vi "SetOutputVoltage_online.vi"() -> ()   [LabVIEW 2018]
uses:
  <vilib>/Utility/error.llb/DialogType.ctl
  <vilib>/DAQmx/write.llb/DAQmx Write (Analog 2D DBL NChan NSamp).vi
  <vilib>/DAQmx/create/channels.llb/DAQmx Create Channel (AO-Voltage-Basic).vi
  <vilib>/DAQmx/configure/timing.llb/DAQmx Timing (Sample Clock).vi
  <vilib>/DAQmx/configure/trigger.llb/DAQmx Start Trigger (Digital Edge).vi
  <vilib>/DAQmx/configure/trigger.llb/DAQmx Start Trigger (Time).vi
  <vilib>/DAQmx/configure/trigger.llb/DAQmx Start Trigger (Analog Edge).vi
  <vilib>/DAQmx/miscellaneous.llb/DAQmx Fill In Error Info.vi
  <resource>/objmgr/daqmx.rc
panel:
  in  "element":dbl=0.1 format="%#_13g"
  in  "Trigger Type":T1(tab)
  in  "Digital Start Trigger Edge":i32(ring)=10280 caption="Edge" items=["Rising"=10280, "Falling"=10171]
  in  "Digital Start Trigger Source":tag="/Dev1/PFI0" caption="Source"
  in  "Digital Pause Trigger Pause When":i32(ring)=10192 caption="Pause When" items=["High"=10192, "Low"=10214]
  in  "Digital Pause Trigger Source":tag="/Dev1/PFI0" caption="Source"
  in  "Analog Start Trigger Level":dbl caption="Level" format="%0.2f"
  in  "Analog Start Trigger Hysteresis":dbl caption="Hysteresis" format="%.2f"
  in  "Analog Start Trigger Slope":i32(ring)=10280 caption="Slope" items=["Rising"=10280, "Falling"=10171]
  in  "Analog Start Trigger Source":string="APFI0" caption="Source"
  in  "Analog Pause Trigger Source":string="APFI0" caption="Source"
  in  "Analog Pause Trigger Pause When":i32(ring)=10093 caption="Pause When" items=["Above Level"=10093, "Below Level"=10107]
  in  "Analog Pause Trigger Level":dbl caption="Level" format="%.2f"
  in  "When":timestamp
  in  "Select Time\nManually":bool
  out "Waveform Graph":waveform(dbl)[](graph)=[{"t0"=timestamp(0 s since 1904-01-01), "dt"=0.001, "Y"=[]}]
  in  "Stop":bool
  in  "Sample Rate":dbl=1000.0
  in  "Sample Clock Source":tag="OnboardClock"
  in  "Max Voltage":dbl=5.0
  in  "Min Voltage":dbl=-5.0
  in  "Physical Channel(s)":tag="Mod2/ao0"
  out "Actual Sample Rate":dbl=1000.0 format="%0.2f"
  # "To enable triggers, select a tab above, and configure the settings.\n\nNot all hardware supports all trigger types. Refer to your device documentation for more information."
  # "This trigger type is not supported in output tasks. \n\nRefer to your device documentation for more information on which triggers are supported."
  # "This trigger type is not supported in output tasks. \n\nRefer to your device documentation for more information on which triggers are supported."
  # "If time is not manually set, task will begin after 10 seconds"
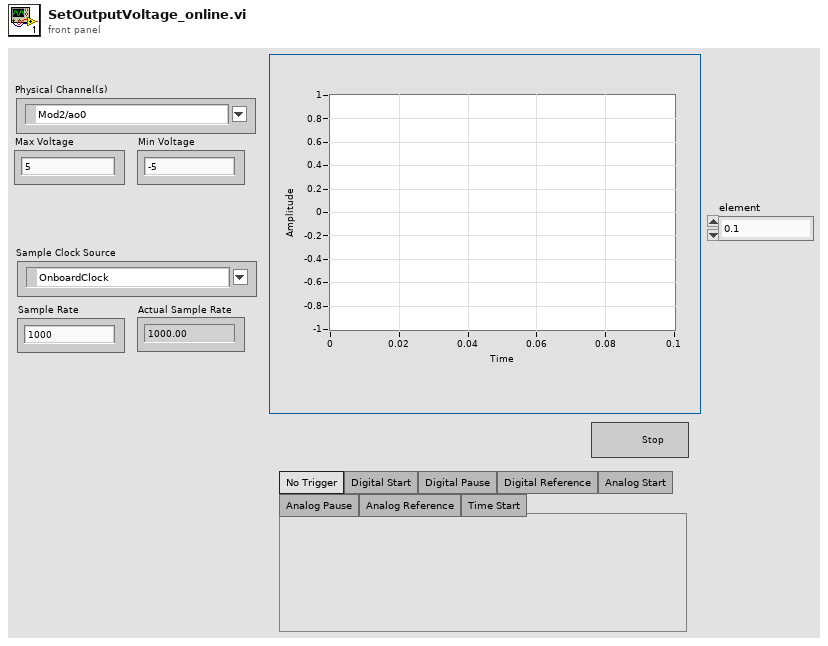
[diagram p1: front panel]
types:
  T1 = enum32{"No Trigger", "Digital Start", "Digital Pause", "Digital Reference", "Analog Start", "Analog Pause", "Analog Reference", "Time Start"}
  T2 = typedef "DialogType.ctl" = u16
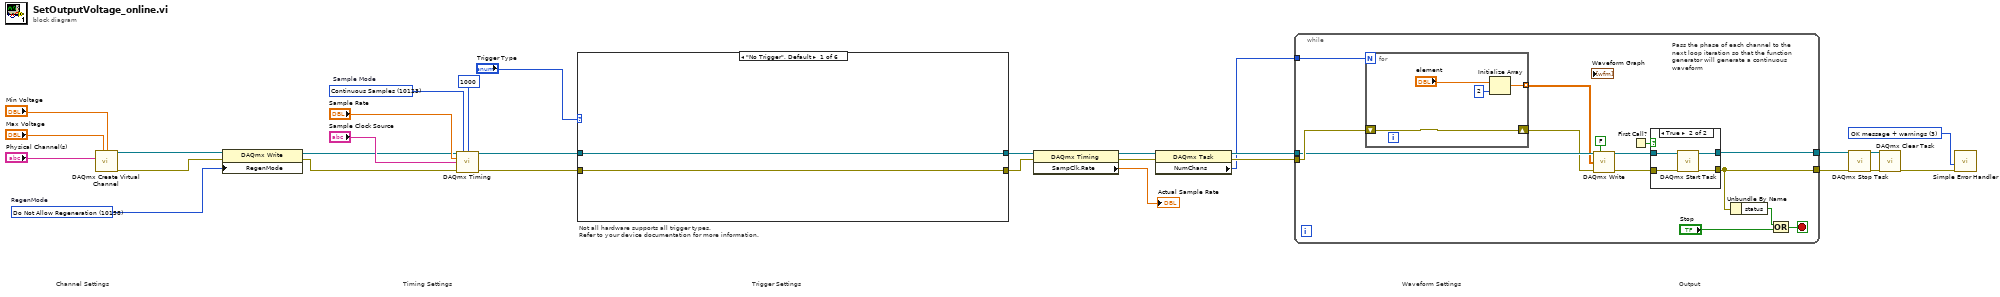
[diagram p0: block diagram]
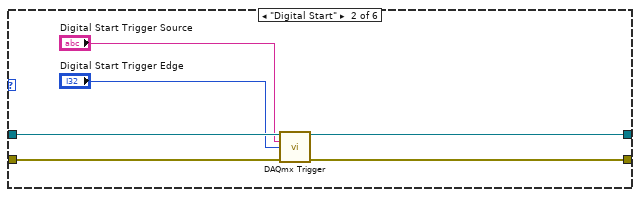
[diagram p3: hidden frame]
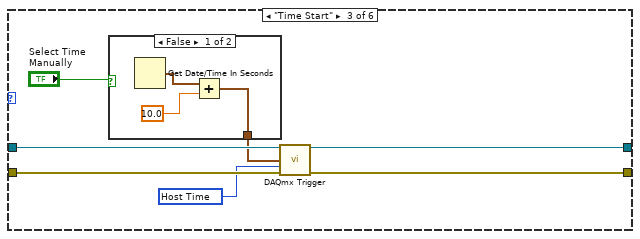
[diagram p4: hidden frame]
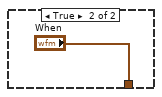
[diagram p5: hidden frame]
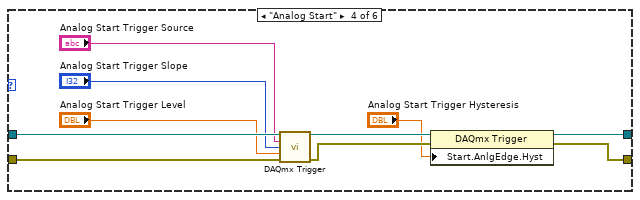
[diagram p6: hidden frame]
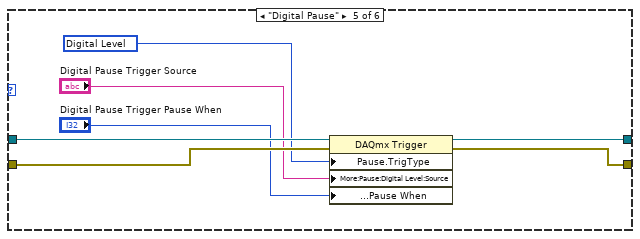
[diagram p7: hidden frame]
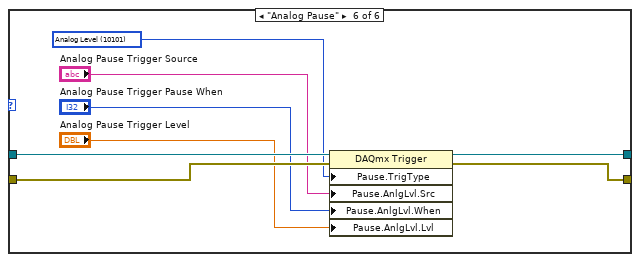
[diagram p8: hidden frame]
diagram:
  w12 = T2 3 items=["no dialog", "OK message", "continue or stop message", "OK message + warnings", "continue/stop + warnings"] ("type of dialog (OK msg:1)")
  w19 = 10158 items=["Allow Regeneration"=10097, "Do Not Allow Regeneration"=10158]  # RegenMode
  w29 = 10123 items=["Finite Samples"=10178, "Continuous Samples"=10123, "Hardware Timed Single Point"=12522]  # Sample Mode
  # "Trigger Settings"
  # "Not all hardware supports all trigger types.\nRefer to your device documentation for more information."
  # "Output"
  # "Waveform Settings"
  # "Timing Settings"
  # "Channel Settings"
  n1 = call-poly <vilib>:"DAQmx Create Virtual Channel.vi"("maximum value"="Max Voltage", "minimum value"="Min Voltage", "physical channels"="Physical Channel(s)") -> ("task out"=w21:refnum<k21>, "error out"=w20:errorcluster)  [unwired: 11 in]
  n2 = property class="DAQmx Write"(reference=w21, error in=w20, "RegenMode"=w19) -> (reference out=w17:refnum<k21>, error out=w18:errorcluster)
  n3 = call-poly <vilib>:"DAQmx Timing.vi"("task/channels in"=w17, "sample mode"=w29, "samples per channel"=1000, "rate"="Sample Rate", "source"="Sample Clock Source", "error in"=w18) -> ("task out"=w5:refnum<k21>, "error out"=w6:errorcluster)  [unwired: 8 in]
  n4 = case shown="\"No Trigger\", Default" "Trigger Type" {
    tunnel: w5 -> [w31 w37 w44 w58 w65 w73]
    tunnel: w6 -> [w30 w36 w43 w57 w62 w70]
    tunnel: [w31 w35 w42 w55 w64 w72] -> w4
    tunnel: [w30 w34 w41 w54 w63 w71] -> w3
    frame "No Trigger", Default {
    }
    frame "Digital Start" {
      n5 = call-poly <vilib>:"DAQmx Trigger.vi"("task/channels in"=w37, "source"="Digital Start Trigger Source", "edge"="Digital Start Trigger Edge", "error in"=w36) -> ("task out"=w35:refnum<k21>, "error out"=w34:errorcluster)  [unwired: 10 in]
    }
    frame "Time Start" {
      w38 = 16126 items=["Host Time"=16126, "I/O Device Time"=16127] ("timescale")
      n6 = case shown="False" "Select Time\nManually" {
        tunnel: [w46 "When"] -> w39
        frame False {
          n7 = Get Date/Time In Seconds() -> (seconds since 1Jan1904=w47:timestamp)
          n8 = Add(x=w47, y=10.0) -> (x+y=w46:timestamp)
        }
        frame True {
        }
      }
      n9 = call-poly <vilib>:"DAQmx Trigger.vi"("task/channels in"=w44, "when"=w39, "timescale"=w38, "error in"=w43) -> ("task out"=w42:refnum<k21>, "error out"=w41:errorcluster)  [unwired: 10 in]
    }
    frame "Analog Start" {
      n10 = call-poly <vilib>:"DAQmx Trigger.vi"("task/channels in"=w58, "source"="Analog Start Trigger Source", "slope"="Analog Start Trigger Slope", "level"="Analog Start Trigger Level", "error in"=w57) -> ("task out"=w53:refnum<k21>, "error out"=w52:errorcluster)  [unwired: 9 in]
      n11 = property class="DAQmx Trigger"(reference=w53, error in=w52, "Start.AnlgEdge.Hyst"="Analog Start Trigger Hysteresis") -> (reference out=w55:refnum<k21>, error out=w54:errorcluster)
    }
    frame "Digital Pause" {
      w61 = 10152 items=["Analog Level"=10101, "Analog Window"=10103, "Digital Level"=10152, "Digital Pattern"=10398, "None"=10230] ("Pause.TrigType")
      n12 = property class="DAQmx Trigger"(reference=w65, error in=w62, "Pause.TrigType"=w61, "More:Pause:Digital Level:Source"="Digital Pause Trigger Source", "More:Pause:Digital Level:Pause When"="Digital Pause Trigger Pause When") -> (reference out=w64:refnum<k21>, error out=w63:errorcluster)
    }
    frame "Analog Pause" {
      w69 = 10101 items=["Analog Level"=10101, "Analog Window"=10103, "Digital Level"=10152, "Digital Pattern"=10398, "None"=10230] ("Pause.TrigType")
      n13 = property class="DAQmx Trigger"(reference=w73, error in=w70, "Pause.TrigType"=w69, "Pause.AnlgLvl.Src"="Analog Pause Trigger Source", "Pause.AnlgLvl.When"="Analog Pause Trigger Pause When", "Pause.AnlgLvl.Lvl"="Analog Pause Trigger Level") -> (reference out=w72:refnum<k21>, error out=w71:errorcluster)
    }
  }
  n14 = property class="DAQmx Timing"(reference=w4, error in=w3) -> (reference out=w9:refnum<k21>, error out=w8:errorcluster, "SampClk.Rate"=→"Actual Sample Rate":dbl)
  n15 = property class="DAQmx Task"(reference=w9, error in=w8) -> (reference out=w11:refnum<k21>, error out=w10:errorcluster, "NumChans"=w2:u32)
  n16 = while {
    tunnel: w10 -> [w87]
    tunnel: w11 -> [w86]
    tunnel: [w81] -> w14
    tunnel: [w80] -> w13
    tunnel: w2 -> [w75]
    stop <- w78 stop-if-true
    # "Pass the phase of each channel to the next loop iteration so that the function generator will generate a continuous waveform"
    n17 = for {
      N: w75 -> [_]
      shift-right: [w97] -> w83
      shift-left: w87 -> [w97]
      tunnel: [w95] -> w74 mode=indexing
      n18 = Initialize Array("element", 2 ("dimension size")) -> (w95:dbl[])
    }
    n19 = call-poly <vilib>:"DAQmx Write.vi"("task/channels in"=w86, "auto start"=FALSE, "data"=w74, "error in"=w83) -> ("task out"=w85:refnum<k21>, "error out"=w84:errorcluster)  [unwired: 9 in, 1 out]
    n20 = First Call?() -> (First Call?: T/F=w82:bool)
    n21 = case shown="True" w82 {
      tunnel: w85 -> [w88 w93]
      tunnel: w84 -> [w89 w92]
      tunnel: [w88 w91] -> w81
      tunnel: [w89 w90] -> w80
      frame False {
      }
      frame True {
        n22 = call <vilib>:"DAQmx Start Task.vi"("task/channels in"=w93, "error in"=w92) -> ("task out"=w91:refnum<k21>, "error out"=w90:errorcluster)  [unwired: 12 in]
      }
    }
    n23 = Unbundle By Name(w80) -> ("status"=w77:bool)
    n24 = Or(x=w77, y="Stop") -> (x .or. y?=w78:bool)
  }
  n25 = call <vilib>:"DAQmx Stop Task.vi"("task/channels in"=w14, "error in"=w13) -> ("task out"=w16:refnum<k21>, "error out"=w15:errorcluster)  [unwired: 12 in]
  n26 = call <vilib>:"DAQmx Clear Task.vi"("task in"=w16, "error in"=w15) -> ("error out"=w28:errorcluster)  [unwired: 13 in]
  n27 = call <vilib>:"Simple Error Handler.vi"("type of dialog (OK msg:1)"=w12, "error in (no error)"=w28) -> ()  [unwired: 3 in, 5 out]
